vi "serialConfigSave.vi"(7 "Ctl":enum16{"read", "write"}(ring), 10 "ViSA Config":T1={"baud rate (9600)"=9600, "flow control (0:none)"=0, "VISA resource name 2"="", "termination char\n(0xA = '\\n' = LF) "=10, "data bits (8)"=8, "parity (0:none)"=enum."None", "timeout (10sec)"=10000, "Enable Termination\nChar (T)"=TRUE, "stop bits (10: 1 bit)"=10} {"stop bits (10: 1 bit)" items=["1.0"=10, "1.5"=15, "2.0"=20]; "data bits (8)" min=5 max=8 step=1; "termination char\n(0xA = '\\n' = LF)" format="%.0x"; "flow control (0:none)" items=["없음", "XON/XOFF", "RTS/CTS", "XON/XOFF & RTS/CTS", "DTR/DSR", "XON/XOFF & DTR/DSR"]}) -> (2 "Reurn":T1={"baud rate (9600)"=9600, "flow control (0:none)"=0, "VISA resource name 2"="", "termination char\n(0xA = '\\n' = LF) "=10, "data bits (8)"=8, "parity (0:none)"=enum."None", "timeout (10sec)"=10000, "Enable Termination\nChar (T)"=TRUE, "stop bits (10: 1 bit)"=10} {"stop bits (10: 1 bit)" items=["1.0"=10, "1.5"=15, "2.0"=20]; "data bits (8)" min=5 max=8 step=1; "termination char\n(0xA = '\\n' = LF)" format="%.0x"; "flow control (0:none)" items=["없음", "XON/XOFF", "RTS/CTS", "XON/XOFF & RTS/CTS", "DTR/DSR", "XON/XOFF & DTR/DSR"]})   [LabVIEW 2023]
uses:
  <vilib>/Utility/config.llb/Write Key (String).vi
  <vilib>/Utility/config.llb/Write Key (U32).vi
  <vilib>/Utility/config.llb/Write Key (I32).vi
  <vilib>/Utility/config.llb/Write Key (Boolean).vi
  <vilib>/Utility/config.llb/Read Key (String).vi
  <vilib>/Utility/config.llb/Read Key (I32).vi
  <vilib>/Utility/config.llb/Read Key (Boolean).vi
  <vilib>/Utility/config.llb/NI_LVConfig.lvlib
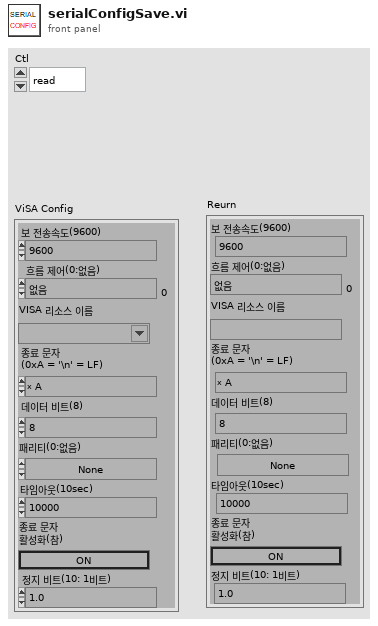
[diagram p1: front panel]
types:
  T1 = cluster{"baud rate (9600)":u32, "flow control (0:none)":u16, "VISA resource name 2":refnum<visa-resource-name>, "termination char\n(0xA = '\\n' = LF) ":u8, "data bits (8)":u16, "parity (0:none)":enum16{"None", "Odd", "Even", "Mark", "Space"}, "timeout (10sec)":u32, "Enable Termination\nChar (T)":bool, "stop bits (10: 1 bit)":u16}
  T2 = typedef "NI_LVConfig.lvlib/Config Data RefNum.ctl" = refnum<k1>
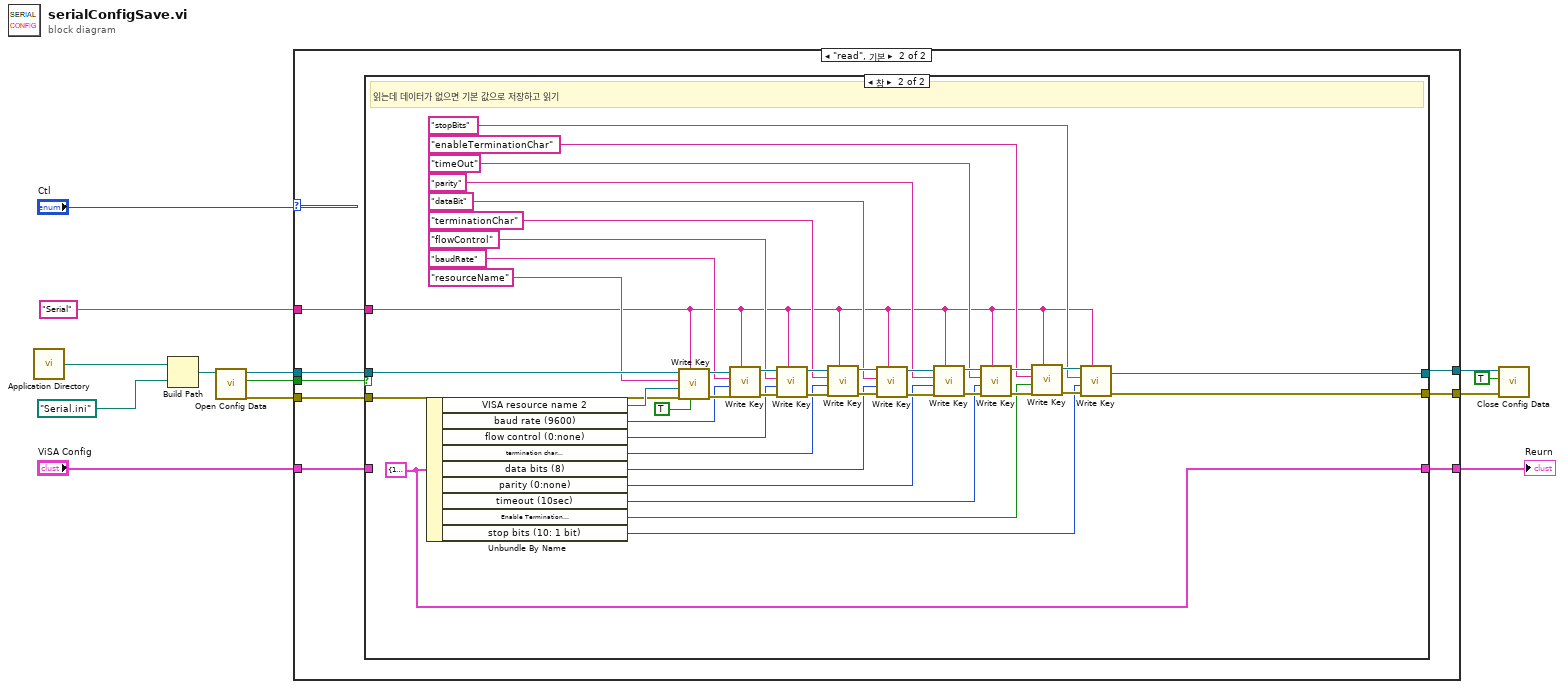
[diagram p0: block diagram]
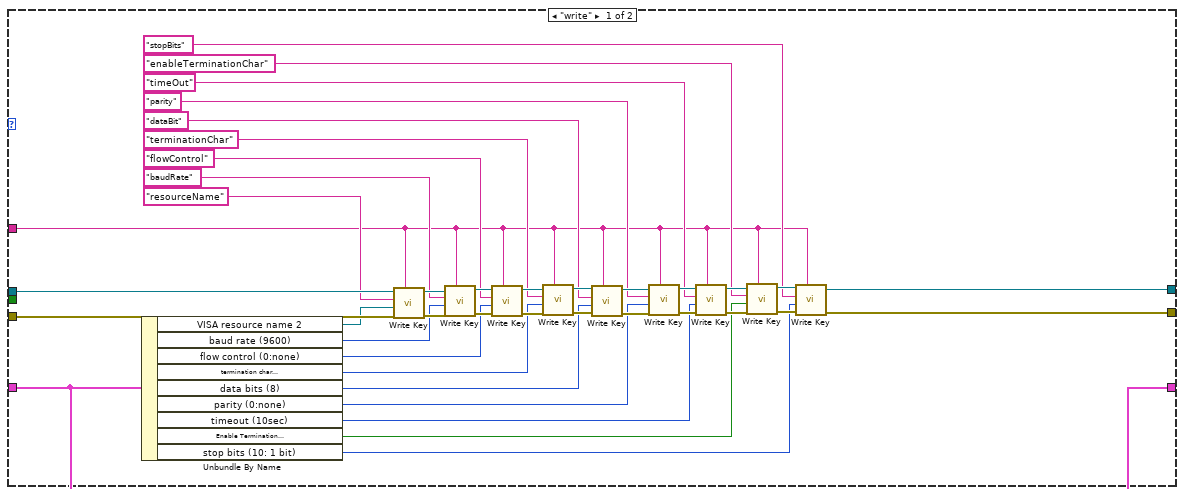
[diagram p2: hidden frame]
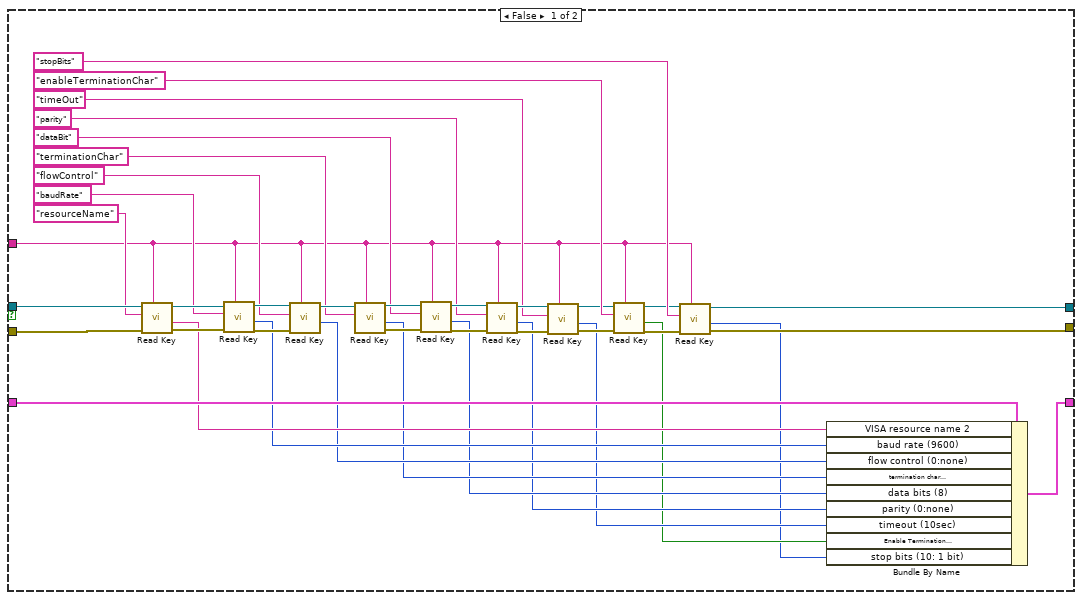
[diagram p3: hidden frame]
diagram:
  n1 = call <vilib>:"Application Directory.vi"() -> ("Application Directory"=w13:path)
  n2 = Build Path(base path=w13, name or relative path=path "Serial.ini" ("이름 또는 상대 경로")) -> (appended path=w11:path)
  n3 = call <vilib>:"Open Config Data.vi"("configuration file path"=w11) -> ("error out"=w6:errorcluster, "file created?"=w10:bool, "refnum"=w9:T2)  [unwired: 8 in]
  n4 = case shown="\"read\", 기본" "Ctl" {
    tunnel: w10 -> [_ w61]
    tunnel: w9 -> [w53 w60]
    tunnel: "ViSA Config" -> [w15 w59]
    tunnel: w6 -> [w52 w58]
    tunnel: [w16 w57] -> w5
    tunnel: [w17 w56] -> w4
    tunnel: [w15 w55] -> w2
    tunnel: "Serial" -> [w14 w54]
    frame "write" {
      n5 = Unbundle By Name(w15) -> ("VISA resource name 2"=w50:refnum<visa-resource-name>, "baud rate (9600)"=w41:u32, "flow control (0:none)"=w40:u16, "termination char\n(0xA = '\\n' = LF)"=w39:u8, "data bits (8)"=w38:u16, "parity (0:none)"=w29:enum16{"None", "Odd", "Even", "Mark", "Space"}, "timeout (10sec)"=w28:u32, "Enable Termination\nChar (T)"=w27:bool, "stop bits (10: 1 bit)"=w26:u16)
      n6 = call-poly <vilib>:"Write Key.vi"("section"=w14, "error in (no error)"=w52, "value"=w50, "key"="resourceName", "refnum"=w53) -> ("error out"=w49:errorcluster, "refnum out"=w48:T2)  [unwired: 4 in, 1 out]
      n7 = call-poly <vilib>:"Write Key.vi"("section"=w14, "error in (no error)"=w49, "value"=w41, "key"="baudRate", "refnum"=w48) -> ("error out"=w47:errorcluster, "refnum out"=w46:T2)  [unwired: 4 in, 1 out]
      n8 = call-poly <vilib>:"Write Key.vi"("section"=w14, "error in (no error)"=w47, "value"=w40, "key"="flowControl", "refnum"=w46) -> ("error out"=w45:errorcluster, "refnum out"=w44:T2)  [unwired: 4 in, 1 out]
      n9 = call-poly <vilib>:"Write Key.vi"("section"=w14, "error in (no error)"=w45, "value"=w39, "key"="terminationChar", "refnum"=w44) -> ("error out"=w43:errorcluster, "refnum out"=w42:T2)  [unwired: 4 in, 1 out]
      n10 = call-poly <vilib>:"Write Key.vi"("section"=w14, "error in (no error)"=w43, "value"=w38, "key"="dataBit", "refnum"=w42) -> ("error out"=w31:errorcluster, "refnum out"=w30:T2)  [unwired: 4 in, 1 out]
      n11 = call-poly <vilib>:"Write Key.vi"("section"=w14, "error in (no error)"=w31, "value"=w29, "key"="parity", "refnum"=w30) -> ("error out"=w32:errorcluster, "refnum out"=w33:T2)  [unwired: 4 in, 1 out]
      n12 = call-poly <vilib>:"Write Key.vi"("section"=w14, "error in (no error)"=w32, "value"=w28, "key"="timeOut", "refnum"=w33) -> ("error out"=w34:errorcluster, "refnum out"=w35:T2)  [unwired: 4 in, 1 out]
      n13 = call-poly <vilib>:"Write Key.vi"("section"=w14, "error in (no error)"=w34, "value"=w27, "key"="enableTerminationChar", "refnum"=w35) -> ("error out"=w36:errorcluster, "refnum out"=w37:T2)  [unwired: 4 in, 1 out]
      n14 = call-poly <vilib>:"Write Key.vi"("section"=w14, "error in (no error)"=w36, "value"=w26, "key"="stopBits", "refnum"=w37) -> ("error out"=w17:errorcluster, "refnum out"=w16:T2)  [unwired: 4 in, 1 out]
    }
    frame "read", Default {
      n15 = case shown="참" w61 {
        tunnel: w60 -> [w101 w142]
        tunnel: w59 -> [w73 _]
        tunnel: [w77 w107] -> w56
        tunnel: [w78 w106] -> w57
        tunnel: w58 -> [w74 w104]
        tunnel: [w72 w105] -> w55
        tunnel: w54 -> [w62 w102]
        frame False {
          n16 = call-poly <vilib>:"Read Key.vi"("section"=w62, "error in (no error)"=w74, "key"="resourceName", "refnum"=w101) -> ("error out"=w98:errorcluster, "value"=w71:string, "refnum out"=w99:T2)  [unwired: 4 in, 1 out]
          n17 = call-poly <vilib>:"Read Key.vi"("section"=w62, "error in (no error)"=w98, "key"="baudRate", "refnum"=w99) -> ("error out"=w94:errorcluster, "value"=w70:i32, "refnum out"=w96:T2)  [unwired: 4 in, 1 out]
          n18 = call-poly <vilib>:"Read Key.vi"("section"=w62, "error in (no error)"=w94, "key"="flowControl", "refnum"=w96) -> ("value"=w69:i32, "refnum out"=w89:T2)  [unwired: 4 in, 2 out]
          n19 = call-poly <vilib>:"Read Key.vi"("section"=w62, "key"="terminationChar", "refnum"=w89) -> ("error out"=w92:errorcluster, "value"=w68:i32, "refnum out"=w88:T2)  [unwired: 5 in, 1 out]
          n20 = call-poly <vilib>:"Read Key.vi"("section"=w62, "error in (no error)"=w92, "key"="dataBit", "refnum"=w88) -> ("error out"=w93:errorcluster, "value"=w67:i32, "refnum out"=w87:T2)  [unwired: 4 in, 1 out]
          n21 = call-poly <vilib>:"Read Key.vi"("section"=w62, "error in (no error)"=w93, "key"="parity", "refnum"=w87) -> ("error out"=w81:errorcluster, "value"=w66:i32, "refnum out"=w86:T2)  [unwired: 4 in, 1 out]
          n22 = call-poly <vilib>:"Read Key.vi"("section"=w62, "error in (no error)"=w81, "key"="timeOut", "refnum"=w86) -> ("error out"=w91:errorcluster, "value"=w65:i32, "refnum out"=w75:T2)  [unwired: 4 in, 1 out]
          n23 = call-poly <vilib>:"Read Key.vi"("section"=w62, "error in (no error)"=w91, "key"="enableTerminationChar", "refnum"=w75) -> ("error out"=w90:errorcluster, "value"=w64:bool, "refnum out"=w76:T2)  [unwired: 4 in, 1 out]
          n24 = call-poly <vilib>:"Read Key.vi"("section"=w62, "error in (no error)"=w90, "key"="stopBits", "refnum"=w76) -> ("error out"=w77:errorcluster, "value"=w63:i32, "refnum out"=w78:T2)  [unwired: 4 in, 1 out]
          n25 = Bundle By Name(cluster=w73, "VISA resource name 2"=w71, "baud rate (9600)"=w70, "flow control (0:none)"=w69, "termination char\n(0xA = '\\n' = LF)"=w68, "data bits (8)"=w67, "parity (0:none)"=w66, "timeout (10sec)"=w65, "Enable Termination\nChar (T)"=w64, "stop bits (10: 1 bit)"=w63) -> (w72:T1)
        }
        frame True {
          w105 = T1 {"baud rate (9600)"=115200, "flow control (0:none)"=0, "VISA resource name 2"="", "termination char\n(0xA = '\\n' = LF) "=0, "data bits (8)"=8, "parity (0:none)"=enum."None", "timeout (10sec)"=10, "Enable Termination\nChar (T)"=FALSE, "stop bits (10: 1 bit)"=0} ("입력 클러스터")
          # "읽는데 데이터가 없으면 기본 값으로 저장하고 읽기"
          n26 = Unbundle By Name(w105) -> ("VISA resource name 2"=w140:refnum<visa-resource-name>, "baud rate (9600)"=w131:u32, "flow control (0:none)"=w130:u16, "termination char\n(0xA = '\\n' = LF)"=w129:u8, "data bits (8)"=w128:u16, "parity (0:none)"=w119:enum16{"None", "Odd", "Even", "Mark", "Space"}, "timeout (10sec)"=w118:u32, "Enable Termination\nChar (T)"=w117:bool, "stop bits (10: 1 bit)"=w116:u16)
          n27 = call-poly <vilib>:"Write Key.vi"("write raw string? (F)"=TRUE, "section"=w102, "error in (no error)"=w104, "value"=w140, "key"="resourceName", "refnum"=w142) -> ("error out"=w139:errorcluster, "refnum out"=w138:T2)  [unwired: 3 in, 1 out]
          n28 = call-poly <vilib>:"Write Key.vi"("section"=w102, "error in (no error)"=w139, "value"=w131, "key"="baudRate", "refnum"=w138) -> ("error out"=w137:errorcluster, "refnum out"=w136:T2)  [unwired: 4 in, 1 out]
          n29 = call-poly <vilib>:"Write Key.vi"("section"=w102, "error in (no error)"=w137, "value"=w130, "key"="flowControl", "refnum"=w136) -> ("error out"=w135:errorcluster, "refnum out"=w134:T2)  [unwired: 4 in, 1 out]
          n30 = call-poly <vilib>:"Write Key.vi"("section"=w102, "error in (no error)"=w135, "value"=w129, "key"="terminationChar", "refnum"=w134) -> ("error out"=w133:errorcluster, "refnum out"=w132:T2)  [unwired: 4 in, 1 out]
          n31 = call-poly <vilib>:"Write Key.vi"("section"=w102, "error in (no error)"=w133, "value"=w128, "key"="dataBit", "refnum"=w132) -> ("error out"=w121:errorcluster, "refnum out"=w120:T2)  [unwired: 4 in, 1 out]
          n32 = call-poly <vilib>:"Write Key.vi"("section"=w102, "error in (no error)"=w121, "value"=w119, "key"="parity", "refnum"=w120) -> ("error out"=w122:errorcluster, "refnum out"=w123:T2)  [unwired: 4 in, 1 out]
          n33 = call-poly <vilib>:"Write Key.vi"("section"=w102, "error in (no error)"=w122, "value"=w118, "key"="timeOut", "refnum"=w123) -> ("error out"=w124:errorcluster, "refnum out"=w125:T2)  [unwired: 4 in, 1 out]
          n34 = call-poly <vilib>:"Write Key.vi"("section"=w102, "error in (no error)"=w124, "value"=w117, "key"="enableTerminationChar", "refnum"=w125) -> ("error out"=w126:errorcluster, "refnum out"=w127:T2)  [unwired: 4 in, 1 out]
          n35 = call-poly <vilib>:"Write Key.vi"("section"=w102, "error in (no error)"=w126, "value"=w116, "key"="stopBits", "refnum"=w127) -> ("error out"=w107:errorcluster, "refnum out"=w106:T2)  [unwired: 4 in, 1 out]
        }
      }
    }
  }
  "Reurn" <- w2
  n36 = call <vilib>:"Close Config Data.vi"("error in (no error)"=w4, "write file if changed (T)"=TRUE, "refnum"=w5) -> ()  [unwired: 7 in, 2 out]
